vi "GetGUID.vi"(0 "Interface in":refnum<class>, 5 "error in (no error)":errorcluster) -> (14 "Interface out":refnum<class>, 15 "GUID":string, 19 "error out":errorcluster)   [LabVIEW 2016, in "GUID Trait With Attributes.lvclass"]
uses:
  GUID Trait With Attributes.lvclass
  GUID Trait With Attributes.lvclass/GUID Trait With Attributes.ctl
panel:
  # "Place Indicators here, and remember\nto connect them to the connector pane"
  # "Place Controls here, and remember\nto connect them to the connector pane"
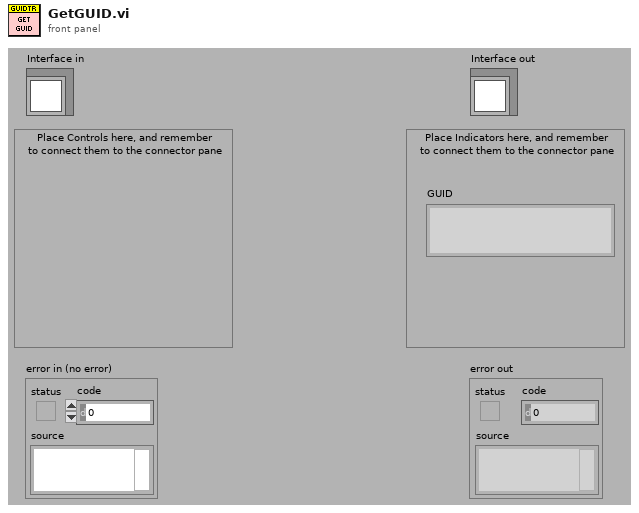
[diagram p1: front panel]
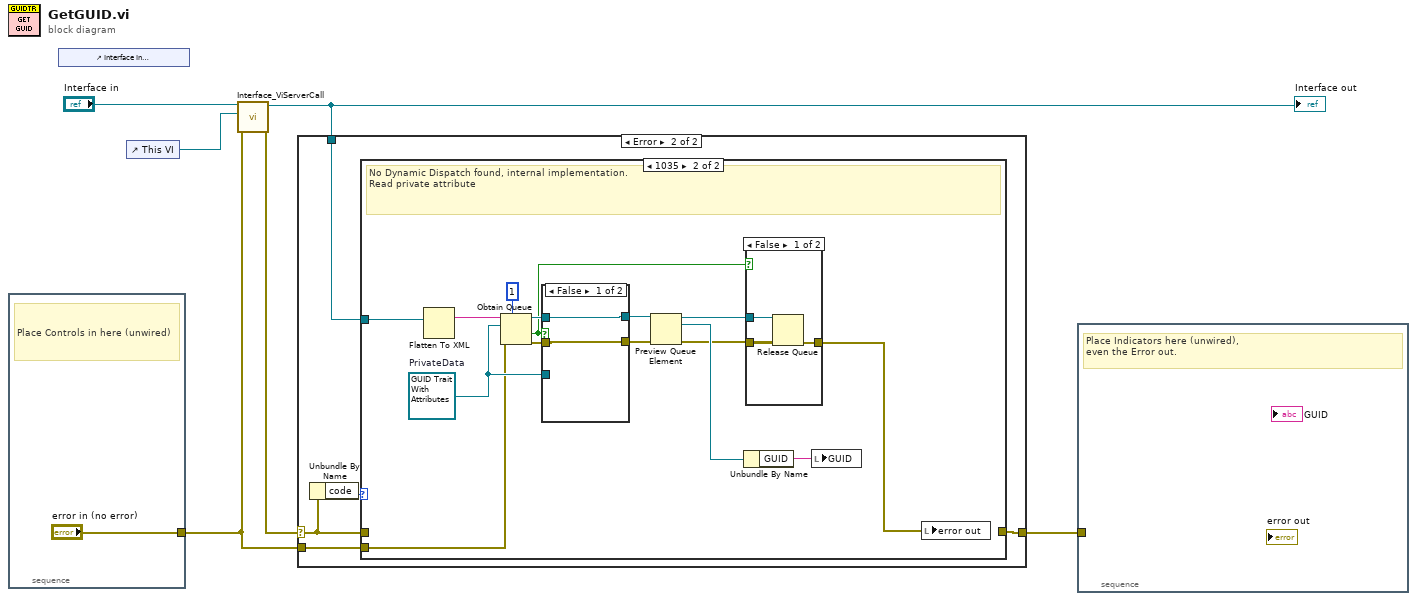
[diagram p0: block diagram]
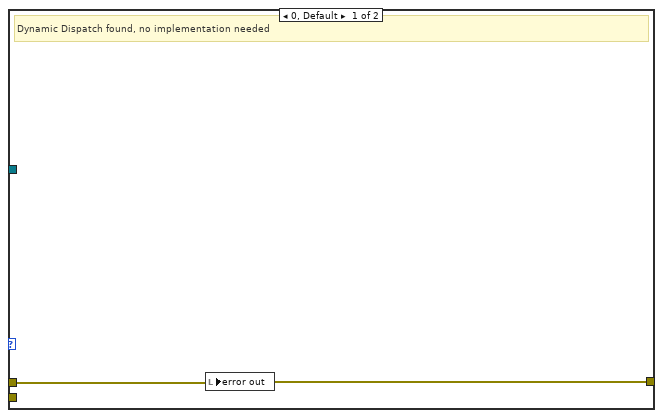
[diagram p3: hidden frame]
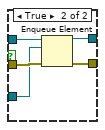
[diagram p5: hidden frame]
diagram:
  n1 = stacked-sequence {
    tunnel: ["error in (no error)"] -> w2
    frame #0 {
      # "Place Controls in here (unwired)"
    }
  }
  n2 = control-ref of="Interface In\nThis reference is needed to make sure this VI's front\npanel isn't removed when building an executable."() -> ()  [unwired: 1 out]
  n3 = control-ref of="This VI"() -> (w5:refnum<vi>)
  n4 = call <vilib>:"Interface_ViServerCall.vi"("error in (no error)"=w2, "Caller VI ref (This is the interface VI's reference)"=w5, "Interface In"="Interface in") -> ("error out"=w4:errorcluster, "Interface Out"=w1:refnum<class>)  [unwired: 7 in]
  "Interface out" <- w1
  n5 = case shown="Error" w4 {
    selector: w4 -> [w8 w13]
    tunnel: [w8 w11] -> w3
    tunnel: w2 -> [_ w10]
    tunnel: w1 -> [_ w9]
    frame No Error {
    }
    frame Error {
      n6 = Unbundle By Name(w13) -> ("code"=w12:i32)
      n7 = case shown="1035" w12 {
        tunnel: w13 -> [w14 _]
        tunnel: [w14 _] -> w11
        tunnel: w10 -> [_ w20]
        tunnel: w9 -> [_ w21]
        frame 0, Default {
          # "Dynamic Dispatch found, no implementation needed"
          n8 = local write "error out"(w14) -> ()
        }
        frame 1035 {
          w26 = refnum<class "GUID Trait With Attributes.lvclass"> refnum  # PrivateData
          # "No Dynamic Dispatch found, internal implementation.\nRead private attribute"
          n9 = Flatten To XML(anything=w21) -> (xml string=w29:string)
          n10 = Obtain Queue(max queue size (-1, unlimited)=1, name (unnamed)=w29, element data type=w26, error in (no error)=w20) -> (queue out=w28:refnum<queue>, created new?=w22:bool, error out=w27:errorcluster)  [unwired: 1 in]
          n11 = case shown="False" w22 {
            tunnel: w28 -> [w34 w40]
            tunnel: w27 -> [w35 w39]
            tunnel: w26 -> [_ w38]
            tunnel: [w34 w37] -> w24
            tunnel: [w35 w36] -> w23
            frame False {
            }
            frame True {
              n12 = Enqueue Element(queue=w40, element=w38, error in (no error)=w39) -> (queue out=w37:refnum<queue>, error out=w36:errorcluster)  [unwired: 1 in, 1 out]
            }
          }
          n13 = Preview Queue Element(queue=w24, error in (no error)=w23) -> (queue out=w15:refnum<queue>, element=w18:refnum<class "GUID Trait With Attributes.lvclass">, error out=w16:errorcluster)  [unwired: 1 in, 1 out]
          n14 = Unbundle By Name(w18) -> ("GUID"=w17:string)
          n15 = case shown="False" w22 {
            tunnel: w15 -> [w32 _]
            tunnel: w16 -> [w31 w33]
            tunnel: [w30 w33] -> w19
            frame False {
              n16 = Release Queue(queue=w32, error in (no error)=w31) -> (error out=w30:errorcluster)  [unwired: 1 in, 2 out]
            }
            frame True {
            }
          }
          n17 = local write "GUID"(w17) -> ()
          n18 = local write "error out"(w19) -> ()
        }
      }
    }
  }
  n19 = stacked-sequence {
    tunnel: w3 -> [_]
    frame #0 {
      # "Place Indicators here (unwired),\neven the Error out."
    }
  }
